vi "Switch Configuration - Scan List Mode - Update UI.vi"(8 "error in (no error)":errorcluster, 11 "Switch Config UI Data In":T1 {"Switch Config Page Item Ref" format="%.0x"}) -> (0 "error out":errorcluster, 3 "Switch Config UI Data Out":T1 {"Switch Config Page Item Ref" format="%.0x"})   [LabVIEW 2015, in "DMM-SWITCH-ScanList System Explorer.lvlib"]
doc: "Enables and disables Scan List controls and indicators depending on Scan List Mode (Automatic/Manual)"
uses:
  DMM-SWITCH-ScanList System Explorer.lvlib
  Configuration Controls/Switch Config VI UI Data.ctl
  Configuration Controls/Switch Config VI UI Ctrl Values.ctl
  Configuration Controls/Switch Config VI UI Ctrl References.ctl
  <instrlib>/niSwitch/niSwitch.LLB/niSwitch Topologies.ctl
  <vilib>/NI Veristand/Custom Device API/Custom Device Item Ref.ctl
  <vilib>/NI Veristand/Custom Device API/Custom Device API.lvlib
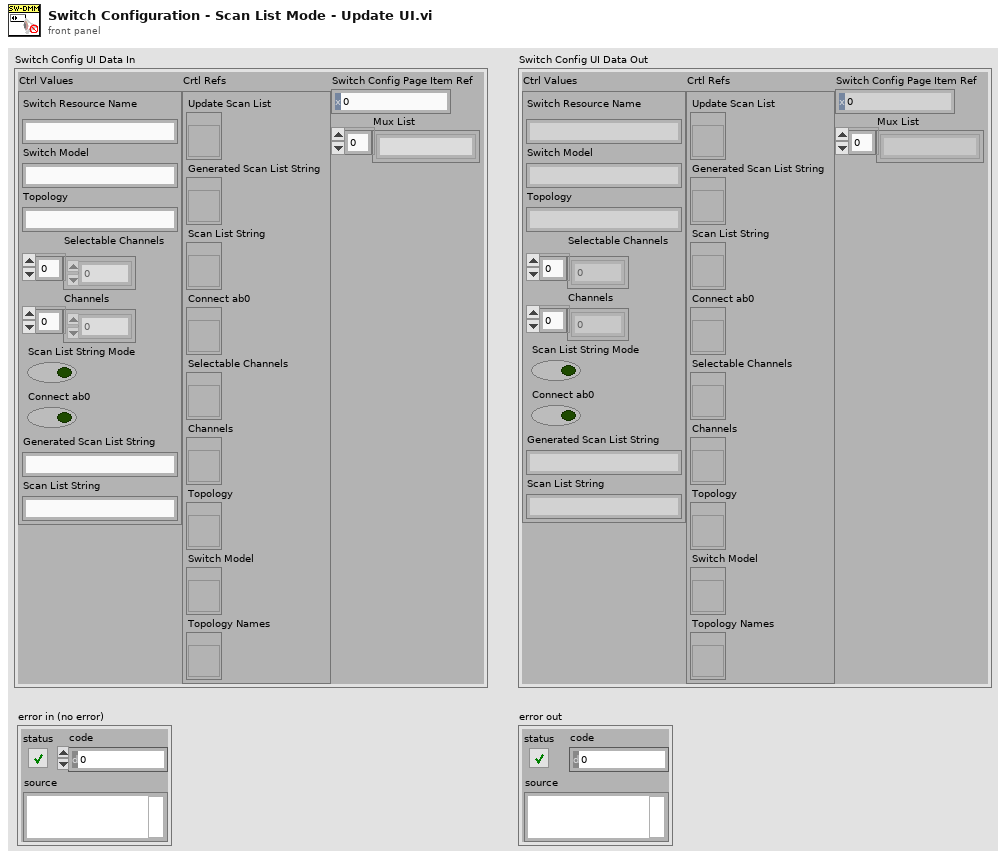
[diagram p1: front panel]
types:
  T1 = typedef "DMM-SWITCH-ScanList System Explorer.lvlib/Switch Config VI UI Data.ctl" = cluster{"Ctrl Values":T2, "Crtl Refs":T3, "Switch Config Page Item Ref":T4, "Mux List":string[]}
  T2 = typedef "DMM-SWITCH-ScanList System Explorer.lvlib/Switch Config VI UI Ctrl Values.ctl" = cluster{"Switch Resource Name":string, "Switch Model":string, "Topology":string, "Selectable Channels":i32[], "Channels":i32[], "Scan List String Mode":bool, "Connect ab0":bool, "Generated Scan List String":string, "Scan List String":string}
  T3 = typedef "DMM-SWITCH-ScanList System Explorer.lvlib/Switch Config VI UI Ctrl References.ctl" = cluster{"Update Scan List":refnum<vi>, "Generated Scan List String":refnum<vi>, "Scan List String":refnum<vi>, "Connect ab0":refnum<vi>, "Selectable Channels":refnum<vi>, "Channels":refnum<vi>, "Topology":refnum<vi>, "Switch Model":refnum<vi>, "Topology Names":refnum<vi>}
  T4 = typedef "Custom Device API.lvlib/Custom Device Item Ref.ctl" = u64
  T5 = enum8{"Enabled", "Disabled", "Disabled and Grayed Out"}
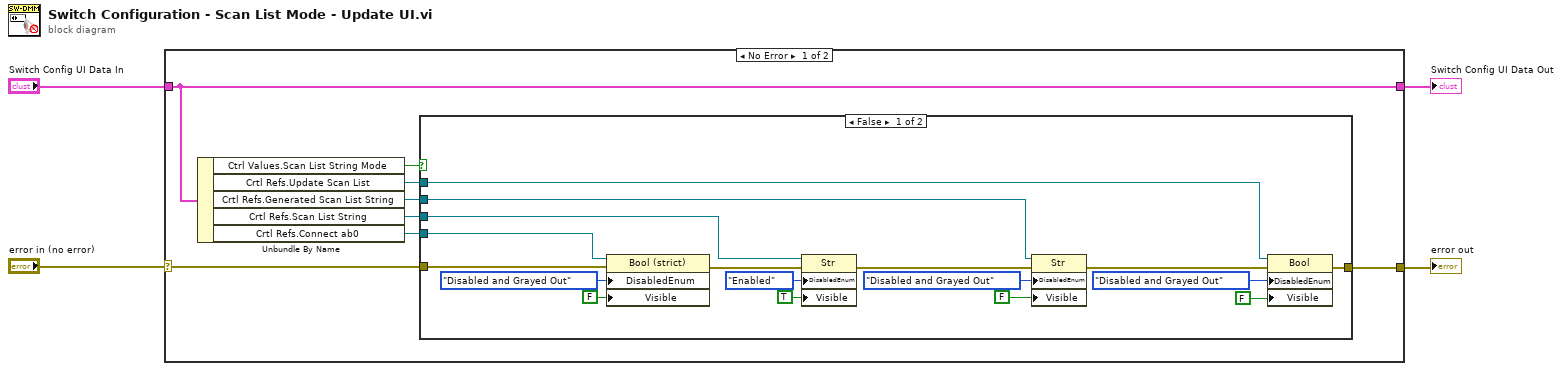
[diagram p0: block diagram]
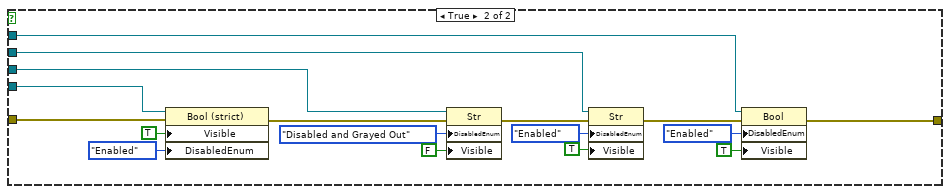
[diagram p2: hidden frame]
diagram:
  n1 = case shown="No Error" "error in (no error)" {
    selector: "error in (no error)" -> [w7 w48]
    tunnel: "Switch Config UI Data In" -> [w5 w47]
    tunnel: [w8 w48] -> w3
    tunnel: [w5 w47] -> w1
    frame No Error {
      n2 = Unbundle By Name(w5) -> ("Ctrl Values.Scan List String Mode"=w6:bool, "Crtl Refs.Update Scan List"=w9:refnum<vi>, "Crtl Refs.Generated Scan List String"=w10:refnum<vi>, "Crtl Refs.Scan List String"=w11:refnum<vi>, "Crtl Refs.Connect ab0"=w12:refnum<vi>)
      n3 = case shown="False" w6 {
        tunnel: w7 -> [w20 w37]
        tunnel: w12 -> [w29 w46]
        tunnel: w11 -> [w28 w45]
        tunnel: [w15 w31] -> w8
        tunnel: w10 -> [w21 w38]
        tunnel: w9 -> [w14 w32]
        frame False {
          n4 = property class="Bool (strict)"(reference=w29, error in=w20, "DisabledEnum"=T5."Disabled and Grayed Out" ("Disabled"), "Visible"=FALSE) -> (error out=w27:errorcluster)  [unwired: 1 out]
          n5 = property class="Str"(reference=w28, error in=w27, "DisabledEnum"=T5."Enabled" ("Disabled"), "Visible"=TRUE) -> (error out=w22:errorcluster)  [unwired: 1 out]
          n6 = property class="Str"(reference=w21, error in=w22, "DisabledEnum"=T5."Disabled and Grayed Out" ("Disabled"), "Visible"=FALSE) -> (error out=w16:errorcluster)  [unwired: 1 out]
          n7 = property class="Bool"(reference=w14, error in=w16, "DisabledEnum"=T5."Disabled and Grayed Out" ("Disabled"), "Visible"=FALSE) -> (error out=w15:errorcluster)  [unwired: 1 out]
        }
        frame True {
          n8 = property class="Bool (strict)"(reference=w46, error in=w37, "Visible"=TRUE, "DisabledEnum"=T5."Enabled" ("Disabled")) -> (error out=w44:errorcluster)  [unwired: 1 out]
          n9 = property class="Str"(reference=w45, error in=w44, "DisabledEnum"=T5."Disabled and Grayed Out" ("Disabled"), "Visible"=FALSE) -> (error out=w39:errorcluster)  [unwired: 1 out]
          n10 = property class="Str"(reference=w38, error in=w39, "DisabledEnum"=T5."Enabled" ("Disabled"), "Visible"=TRUE) -> (error out=w33:errorcluster)  [unwired: 1 out]
          n11 = property class="Bool"(reference=w32, error in=w33, "DisabledEnum"=T5."Enabled" ("Disabled"), "Visible"=TRUE) -> (error out=w31:errorcluster)  [unwired: 1 out]
        }
      }
    }
    frame Error {
    }
  }
  "error out" <- w3
  "Switch Config UI Data Out" <- w1
